vi "Watt Transducer.vi"(8 "Compressor Type":string(combo), 10 "RPM":dbl, 11 "Array in":dbl[](array[numeric])) -> (3 "Array out":dbl[](array[numeric]))   [LabVIEW 2017]
doc: "Reads the input from the watt transducer"
panel:
  in  "input variable 8":dbl=-27.5 format="%#_13g"
  in  "input variable 7":dbl=6.875 format="%#_13g"
  out "AI2":dbl
  in  "input variable 6":dbl format="%#_13g"
  in  "input variable 5":dbl=100.02 format="%#_13g"
  out "kW":dbl
  out "kVAR":dbl
  in  "input variable 4":dbl=-27.5 format="%#_13g"
  in  "input variable 3":dbl=6.875 format="%#_13g"
  in  "input variable 2":dbl=-27.5 format="%#_13g"
  in  "input variable":dbl=6.875 format="%#_13g"
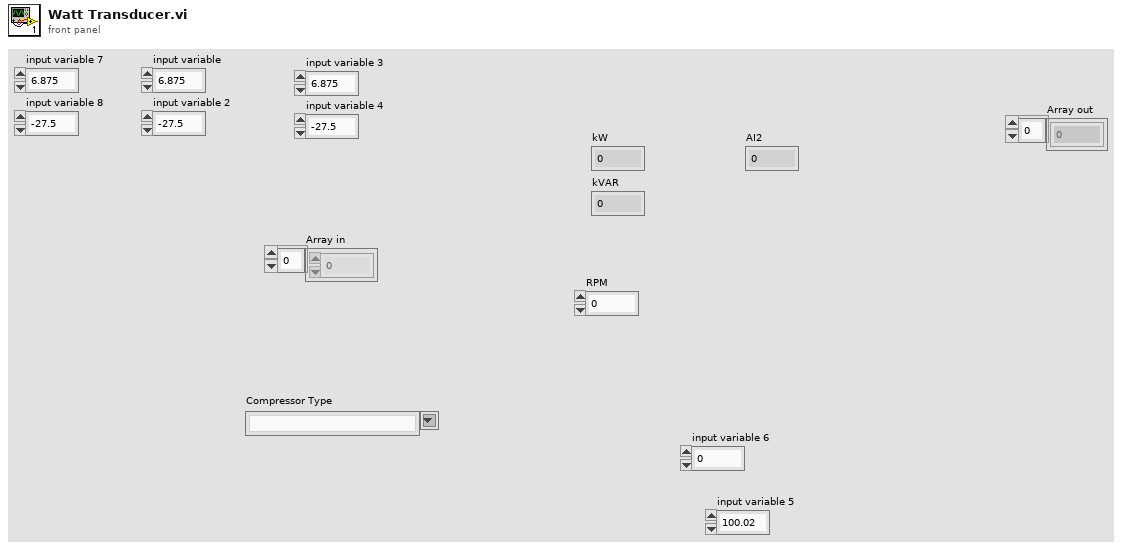
[diagram p1: front panel]
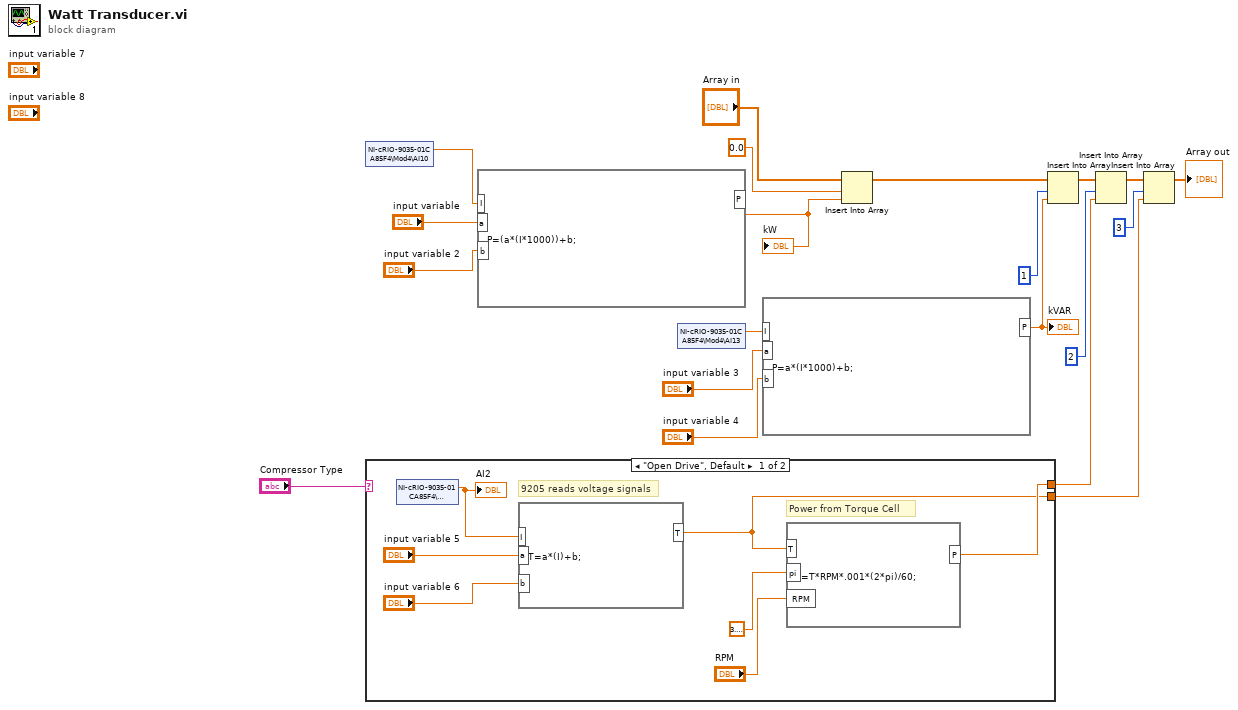
[diagram p0: block diagram]
diagram:
  n1 = shared-variable "NI-cRIO-9035-01CA85F4\\Mod4\\AI10"() -> (w9:dbl)  [unwired: 1 in, 1 out]
  n2 = case shown="\"Open Drive\", Default" "Compressor Type" {
    tunnel: [w23 _] -> w7
    tunnel: [w22 _] -> w4
    frame "Open Drive", Default {
      # "Power from Torque Cell"
      # "9205 reads voltage signals"
      n3 = shared-variable "NI-cRIO-9035-01CA85F4\\EtherCAT Master\\Device\\Mod1\\AI2"() -> (w21:dbl)  [unwired: 1 in, 1 out]
      "AI2" <- w21
      n4 = formula code="T=a*(I)+b;"("I"=w21, "a"="input variable 5", "b"="input variable 6") -> ("T"=w22:dbl)
      n5 = formula code="P=T*RPM*.001*(2*pi)/60;"("T"=w22, "RPM"="RPM", "pi"=3.141592653589793) -> ("P"=w23:dbl)
    }
    frame "Hermetic/Semi-hermetic" {
    }
  }
  n6 = formula code="P=(a*(I*1000))+b;"("I"=w9, "a"="input variable", "b"="input variable 2") -> ("P"=w12:dbl)
  "kW" <- w12
  n7 = shared-variable "NI-cRIO-9035-01CA85F4\\Mod4\\AI13"() -> (w15:dbl)  [unwired: 1 in, 1 out]
  n8 = formula code="P=a*(I*1000)+b;"("I"=w15, "a"="input variable 3", "b"="input variable 4") -> ("P"=w8:dbl)
  "kVAR" <- w8
  n9 = Insert Into Array(array="Array in", index=0.0 ("new element/subarray"), new element=w12) -> (w18:dbl[])
  n10 = Insert Into Array(array=w18, index=1, new element=w8) -> (w5:dbl[])
  n11 = Insert Into Array(array=w5, index=2, new element=w7) -> (w2:dbl[])
  n12 = Insert Into Array(array=w2, index=3, new element=w4) -> (→"Array out":dbl[])
